vi "EVT HLP Set Image IMAQ Buffer Gray Scale U8.vi"(6 "widthLV":i32, 7 "height":i32, 9 "width":i32, 10 "srcBuffer":i64, 11 "IMAQbuffer":i64) -> ()   [LabVIEW 2019, in "EmergentCameraC.lvlib"]
doc: "EMERGENTCAMERAC_API void EVT_HLP_SetImageIMAQBuffer_GrayScaleU8(UCHAR_PTR IMAQbuffer, UCHAR_PTR srcBuffer, int width, int height, int widthLV);"
uses:
  EmergentCameraC.lvlib
  emergentInstall_Windows/win64/eSDK/bin/EmergentCameraC.dll
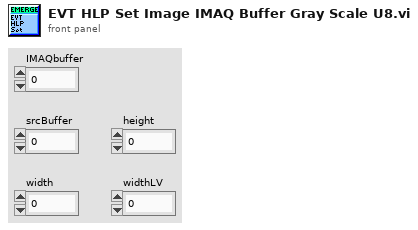
[diagram p1: front panel]
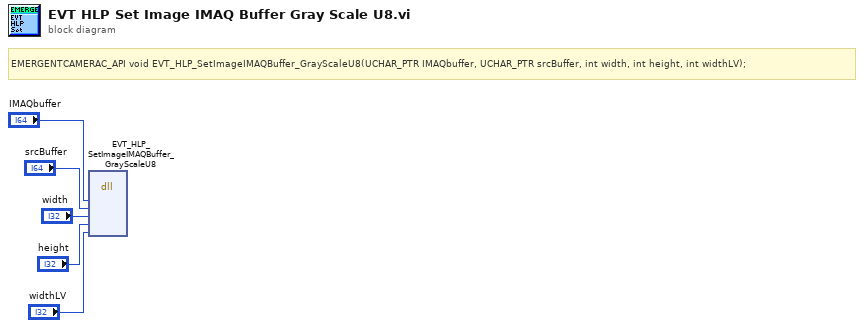
[diagram p0: block diagram]
diagram:
  # "EMERGENTCAMERAC_API void EVT_HLP_SetImageIMAQBuffer_GrayScaleU8(UCHAR_PTR IMAQbuffer, UCHAR_PTR srcBuffer, int width, int height, int widthLV);"
  n1 = dll-call lib="E:/emergent/host-new_QT/emergentInstall_Windows/win64/eSDK/bin/EmergentCameraC.*" fn="EVT_HLP_SetImageIMAQBuffer_GrayScaleU8"("IMAQbuffer"="IMAQbuffer", "srcBuffer"="srcBuffer", "width"="width", "height"="height", "widthLV"="widthLV") -> ()  [unwired: 9 in, 2 out]
